vi "saveLogEntry.vi"(8 "error in (no error)":errorcluster, 11 "Logger in":refnum<class "Log.lvclass">) -> (0 "error out":errorcluster, 3 "Logger out":refnum<class "Log.lvclass">)   [LabVIEW 2013, in "Log.lvlib" / "Log.lvclass"]
uses:
  <userlib>/Common/Log/Log/Log.lvclass
  <userlib>/Common/Log/Log/Log.lvclass/Log.ctl
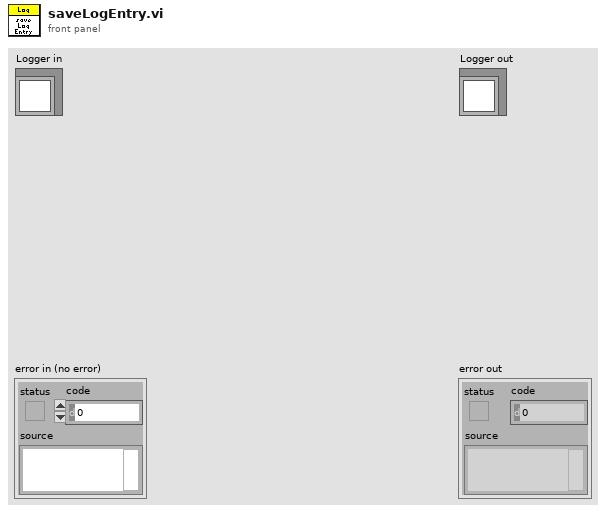
[diagram p1: front panel]
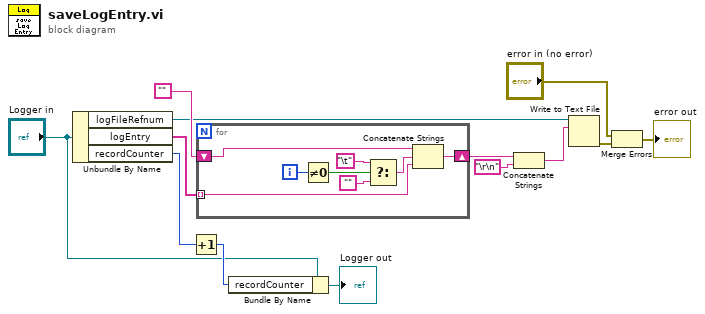
[diagram p0: block diagram]
diagram:
  n1 = Unbundle By Name("Logger in") -> ("logFileRefnum"=w4:refnum<file>, "logEntry"=w9:string[], "recordCounter"=w13:u32)
  n2 = Increment(x=w13) -> (x+1=w12:u32)
  n3 = for {
    tunnel: w9 -> [w16] mode=indexing
    shift-right: [w15] -> w6
    shift-left: "" -> [w20]
    i -> [w21]
    n4 = Not Equal To 0?(x=w21) -> (x != 0?=w19:bool)
    n5 = Select(t="\t", s=w19, f="") -> (s? t:f=w14:string)
    n6 = Concatenate Strings(w20, w14, w16) -> (w15:string)
  }
  n7 = Bundle By Name(cluster="Logger in", "recordCounter"=w12) -> (→"Logger out":refnum<class "Log.lvclass">)
  n8 = Concatenate Strings(w6, "\r\n") -> (w5:string)
  n9 = Write to Text File(file (use dialog)=w4, text=w5) -> (error out=w2:errorcluster)  [unwired: 2 in, 2 out]
  n10 = Merge Errors("error in (no error)", w2) -> (→"error out":errorcluster)
